vi "WriteConfigFiles.vi"(8 "error in":errorcluster, 11 "variant in":variant) -> (0 "error out":errorcluster, 3 "variant out":variant)   [LabVIEW 2013]
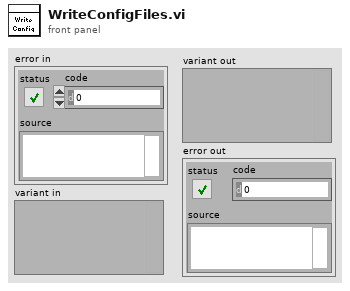
[diagram p1: front panel]
types:
  T1 = enum16{"open", "replace", "create", "open or create", "replace or create", "replace or create with confirmation"}
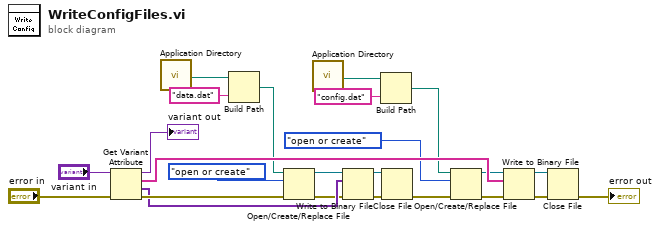
[diagram p0: block diagram]
diagram:
  n1 = Get Variant Attribute(Variant="variant in", error in="error in") -> (duplicate Variant=→"variant out":variant, names=w19:string[], values=w10:variant[], error out=w20:errorcluster)  [unwired: 2 in]
  n2 = call <vilib>:"Application Directory.vi"() -> ("Application Directory"=w9:path)
  n3 = Build Path(base path=w9, name or relative path="data.dat") -> (appended path=w3:path)
  n4 = Open/Create/Replace File(file path (use dialog)=w3, error in=w20, operation (0:open)=T1."open or create") -> (refnum out=w4:refnum<file>, error out=w7:errorcluster)  [unwired: 3 in, 1 out]
  n5 = call <vilib>:"Application Directory.vi"() -> ("Application Directory"=w11:path)
  n6 = Write to Binary File(file (use dialog)=w4, data=w10, error in=w7) -> (refnum out=w6:refnum<file>, error out=w8:errorcluster)  [unwired: 3 in, 1 out]
  n7 = Build Path(base path=w11, name or relative path="config.dat") -> (appended path=w17:path)
  n8 = Close File(refnum=w6, error in=w8) -> (error out=w21:errorcluster)  [unwired: 1 out]
  n9 = Open/Create/Replace File(file path (use dialog)=w17, error in=w21, operation (0:open)=T1."open or create") -> (refnum out=w16:refnum<file>, error out=w13:errorcluster)  [unwired: 3 in, 1 out]
  n10 = Write to Binary File(file (use dialog)=w16, data=w19, error in=w13) -> (refnum out=w14:refnum<file>, error out=w12:errorcluster)  [unwired: 3 in, 1 out]
  n11 = Close File(refnum=w14, error in=w12) -> (error out=→"error out":errorcluster)  [unwired: 1 out]
